vi "5492_WPI_RobotDriveOpen6MotorWithTalonSRX.vi"(0 "Front Left Motor":T1=enum."Invalid", 1 "Front Right Motor":T1=enum."Invalid", 2 "Back Left Motor":T1=enum."Invalid", 3 "Back Right Motor":T1=enum."Invalid", 4 "Middle Left Motor":T1=enum."Invalid", 5 "Middle Right Motor":T1=enum."Invalid", 7 "error in (no error)":errorcluster, 8 "Front Left Motor Inverted":bool, 9 "Middle Left Motor Inverted":bool, 10 "Back Left Motor Inverted":bool, 15 "Back Right Motor Inverted":bool, 16 "Front Right Motor Inverted":bool, 17 "Middle Right Motor Inverted":bool) -> (20 "RobotDriveDevRef":T2={"DevStatus"={"status"=FALSE, "code"=0, "source"=""}, "Motors[]"=[], "Square Inputs"=FALSE, "Max Output"=1.0}, 27 "error out":errorcluster)   [LabVIEW 2016]
doc: "Opens a reference to the robot drive for a two-motor robot using TalonSRX motor controllers.\n\nThis software is licensed. Open the labview\\readme\\WPI Robotics Library Open Source License.txt file for more information."
uses:
  <vilib>/Rock Robotics/SystemInterfaces/DIO/FPGA_DIOPWMChannel.ctl
  <vilib>/Rock Robotics/WPI/RobotDrive/WPI_RobotDriveDevRef.ctl
  <vilib>/Rock Robotics/WPI/MotorControl/WPI_MotorControlDeviceRef.ctl
  <vilib>/Rock Robotics/WPI/MotorControl/WPI_MotorControlType.ctl
  <vilib>/Rock Robotics/WPI/PWM/WPI_PWMDeadband.ctl
  <vilib>/Rock Robotics/WPI/SafetyOutput/WPI_SafetyOutputConfigMenu.ctl
  <vilib>/Rock Robotics/WPI/ThirdParty/CanMotor/TalonSRX/WPI_CANTalonSRX_APIControlMode.ctl
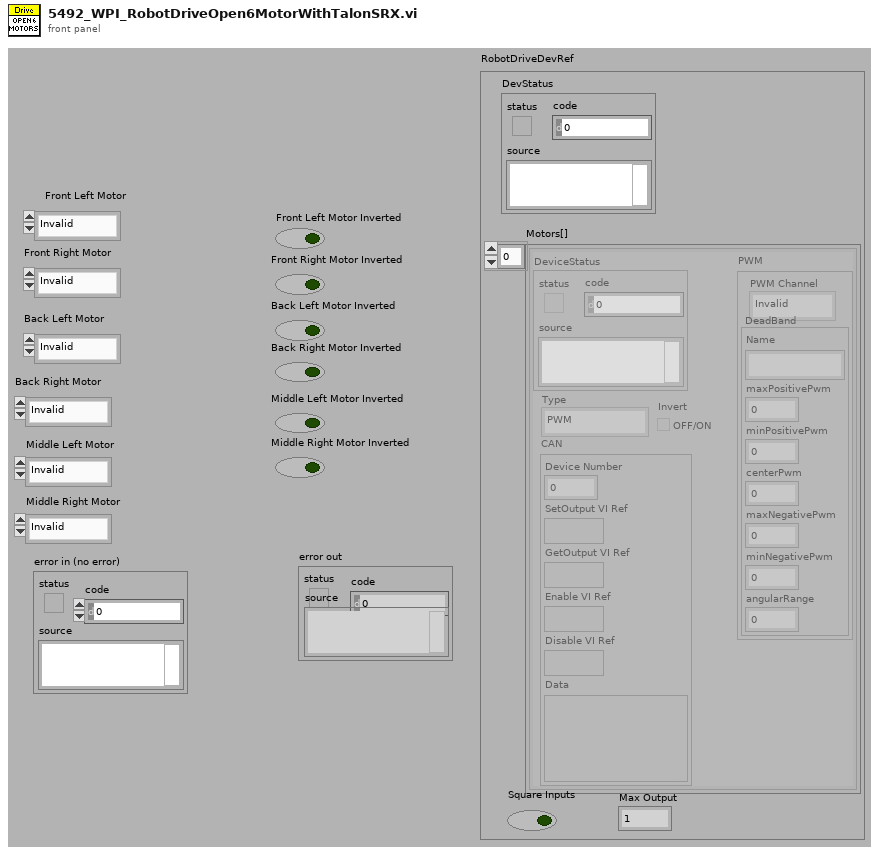
[diagram p1: front panel]
types:
  T1 = typedef "FPGA_DIOPWMChannel.ctl" = enum8{"PWM 0", "PWM 1", "PWM 2", "PWM 3", "PWM 4", "PWM 5", "PWM 6", "PWM 7", "PWM 8", "PWM 9", "PWM MXP 0", "PWM MXP 1", "PWM MXP 2", "PWM MXP 3", "PWM MXP 4", "PWM MXP 5", "PWM MXP 6", "PWM MXP 7", "PWM MXP 8", "PWM MXP 9", "Invalid"}
  T2 = typedef "WPI_RobotDriveDevRef.ctl" = cluster{"DevStatus":errorcluster, "Motors[]":T3[], "Square Inputs":bool, "Max Output":dbl}
  T3 = typedef "WPI_MotorControlDeviceRef.ctl" = cluster{"DeviceStatus":errorcluster, "Type":T4, "PWM":cluster{"PWM Channel":T1, "DeadBand":T5}, "CAN":cluster{"Device Number":u8, "SetOutput VI Ref":variant, "GetOutput VI Ref":variant, "Enable VI Ref":variant, "Disable VI Ref":variant, "Data":variant}, "Invert":bool}
  T4 = typedef "WPI_MotorControlType.ctl" = enum16{"PWM", "CAN"}
  T5 = typedef "WPI_PWMDeadband.ctl" = cluster{"Name":string, "maxPositivePwm":i32, "minPositivePwm":i32, "centerPwm":i32, "maxNegativePwm":i32, "minNegativePwm":i32, "angularRange":u16}
  T6 = typedef "WPI_CANTalonSRX_APIControlMode.ctl" = enum8{"Percent VBus", "Speed", "Position", "Slave", "Unchanged / Invalid", "Voltage Compensation", "Current", "Motion Profile", "Motion Magic"}
  T7 = typedef "WPI_SafetyOutputConfigMenu.ctl" = enum16{"Enable", "Disable"}
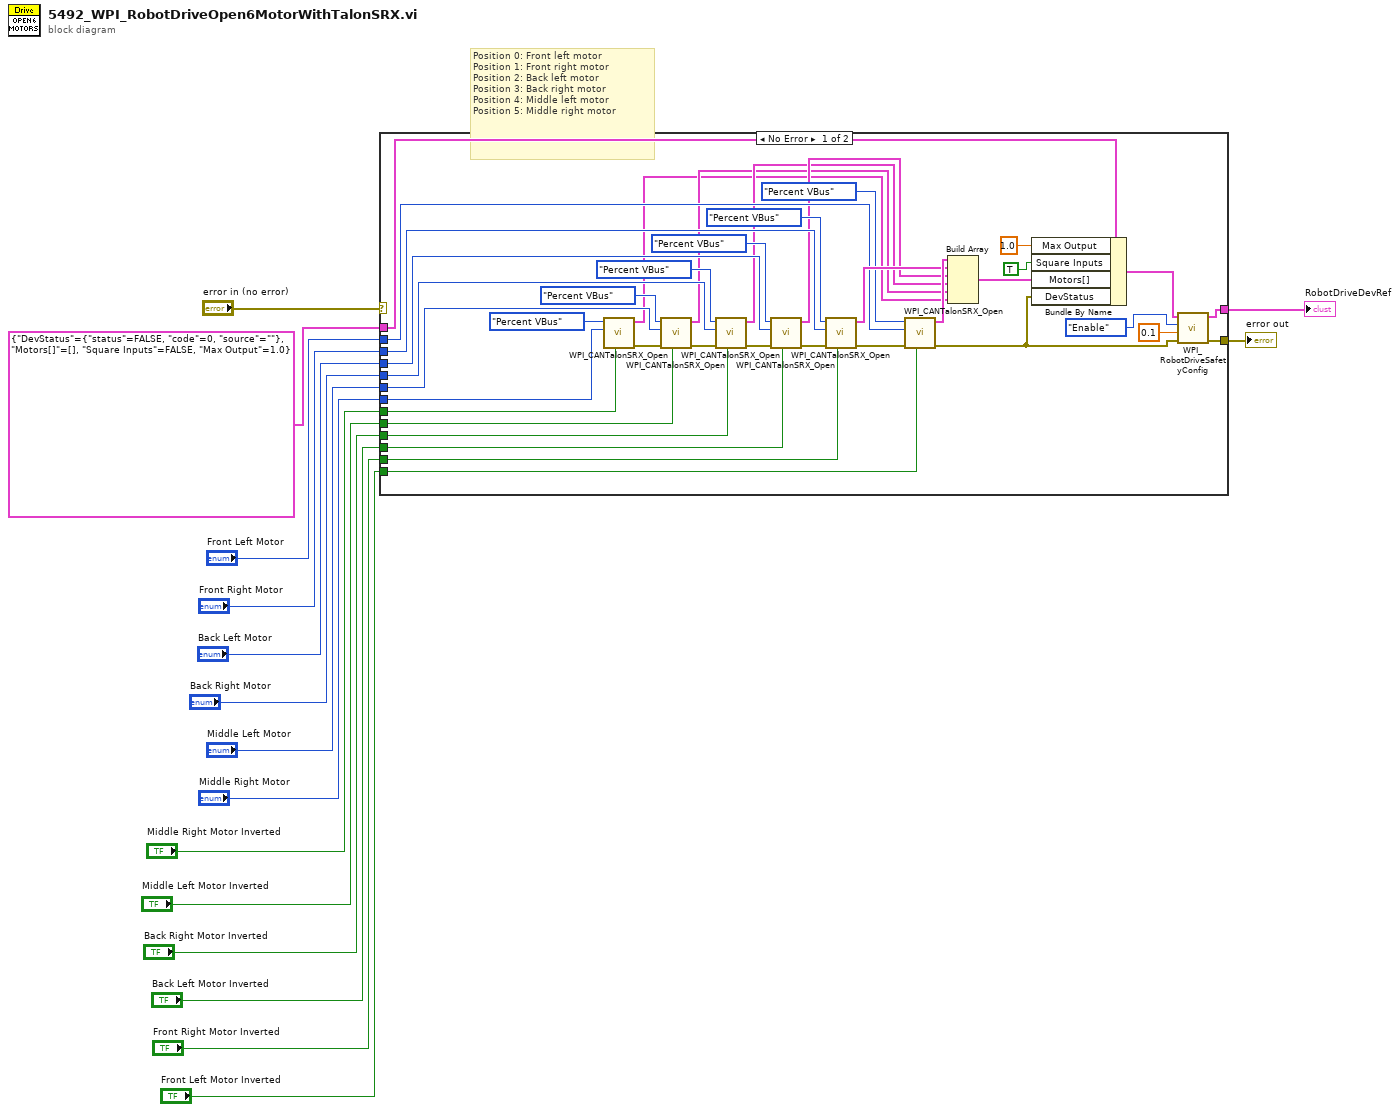
[diagram p0: block diagram]
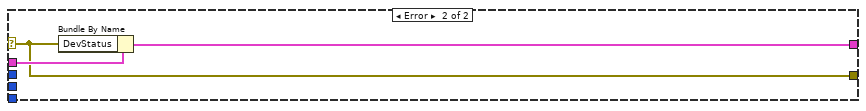
[diagram p2: hidden frame]
diagram:
  # "Position 0: Front left motor\nPosition 1: Front right motor\nPosition 2: Back left motor\nPosition 3: Back right motor\nPosition 4: Middle left motor\nPosition 5: Middle right motor"
  n1 = case shown="No Error" "error in (no error)" {
    selector: "error in (no error)" -> [_ w56]
    tunnel: "Front Left Motor" -> [w37 _]
    tunnel: "Front Right Motor" -> [w35 _]
    tunnel: [w43 w58] -> w9
    tunnel: "Front Left Motor Inverted" -> [w49 _]
    tunnel: "Front Right Motor Inverted" -> [w50 _]
    tunnel: T2 {"DevStatus"={"status"=FALSE, "code"=0, "source"=""}, "Motors[]"=[], "Square Inputs"=FALSE, "Max Output"=1.0} ("RobotDriveDevRef") -> [w54 w57]
    tunnel: [w44 w56] -> w11
    tunnel: "Middle Left Motor" -> [w33 _]
    tunnel: "Middle Right Motor" -> [w31 _]
    tunnel: "Middle Left Motor Inverted" -> [w40 _]
    tunnel: "Middle Right Motor Inverted" -> [w39 _]
    tunnel: "Back Left Motor" -> [w27 _]
    tunnel: "Back Left Motor Inverted" -> [w26 _]
    tunnel: "Back Right Motor" -> [w25 _]
    tunnel: "Back Right Motor Inverted" -> [w24 _]
    frame No Error {
      n2 = call <vilib>:"WPI_CANTalonSRX_Open.vi"("Invert"=w39, "Device Number"=w31, "Control Mode"=WPI_CANTalonSRX_APIControlMode."Percent VBus") -> ("error out"=w38:errorcluster, "CAN Talon SRX Ref"=w17:T3)  [unwired: 7 in]
      n3 = call <vilib>:"WPI_CANTalonSRX_Open.vi"("Invert"=w40, "error in"=w38, "Device Number"=w33, "Control Mode"=WPI_CANTalonSRX_APIControlMode."Percent VBus") -> ("error out"=w23:errorcluster, "CAN Talon SRX Ref"=w18:T3)  [unwired: 6 in]
      n4 = call <vilib>:"WPI_CANTalonSRX_Open.vi"("Invert"=w24, "error in"=w23, "Device Number"=w25, "Control Mode"=WPI_CANTalonSRX_APIControlMode."Percent VBus") -> ("error out"=w22:errorcluster, "CAN Talon SRX Ref"=w19:T3)  [unwired: 6 in]
      n5 = call <vilib>:"WPI_CANTalonSRX_Open.vi"("Invert"=w26, "error in"=w22, "Device Number"=w27, "Control Mode"=WPI_CANTalonSRX_APIControlMode."Percent VBus") -> ("error out"=w21:errorcluster, "CAN Talon SRX Ref"=w20:T3)  [unwired: 6 in]
      n6 = call <vilib>:"WPI_CANTalonSRX_Open.vi"("Invert"=w50, "error in"=w21, "Device Number"=w35, "Control Mode"=WPI_CANTalonSRX_APIControlMode."Percent VBus") -> ("error out"=w53:errorcluster, "CAN Talon SRX Ref"=w51:T3)  [unwired: 6 in]
      n7 = call <vilib>:"WPI_CANTalonSRX_Open.vi"("Invert"=w49, "error in"=w53, "Device Number"=w37, "Control Mode"=WPI_CANTalonSRX_APIControlMode."Percent VBus") -> ("error out"=w45:errorcluster, "CAN Talon SRX Ref"=w52:T3)  [unwired: 6 in]
      n8 = Build Array(w52, w51, w20, w19, w18, w17) -> (w55:T3[])
      n9 = Bundle By Name(cluster=w54, "Max Output"=1.0, "Square Inputs"=TRUE, "Motors[]"=w55, "DevStatus"=w45) -> (w47:T2)
      n10 = call <vilib>:"WPI_RobotDriveSafetyConfig.vi"("error in (no error)"=w45, "timeout (s)"=0.1, "mode"=WPI_SafetyOutputConfigMenu."Enable", "RobotDriveDevRef"=w47) -> ("error out"=w44:errorcluster, "RobotDriveDevRef"=w43:T2)  [unwired: 6 out]
    }
    frame Error {
      n11 = Bundle By Name(cluster=w57, "DevStatus"=w56) -> (w58:T2)
    }
  }
  "RobotDriveDevRef" <- w9
  "error out" <- w11
